vi "Write ID.vi"(8 "error in (no error)":errorcluster, 10 "ID":u8, 11 "Channel in":refnum<class "Channel.lvclass">) -> (0 "error out":errorcluster, 3 "Channel out":refnum<class "Channel.lvclass">)   [LabVIEW 2018, in "Channel.lvclass"]
uses:
  Channel.lvclass
  Channel.lvclass/Channel.ctl
  Save Image/Save Image.lvclass/Save Image.ctl
  Save Image/Save Image.lvclass
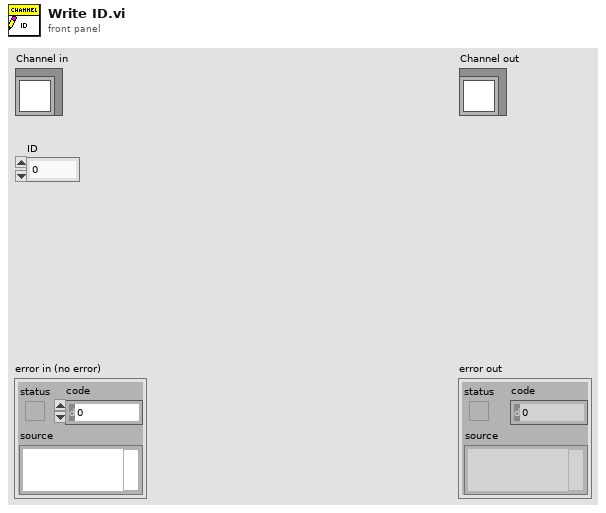
[diagram p1: front panel]
types:
  T1 = cluster{"COMNENT":string, "OBSTYPE":string, "ACSVRSN":string, "CHANNEL":u16, "LAST_IMG_NAME":string, "NIGHTDIR":string}
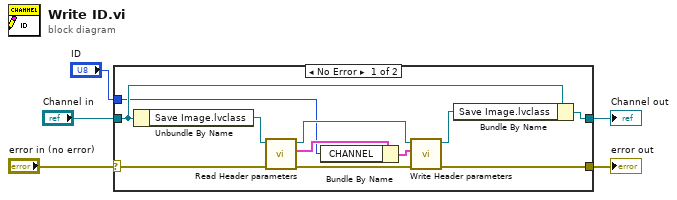
[diagram p0: block diagram]
diagram:
  n1 = case shown="No Error" "error in (no error)" {
    selector: "error in (no error)" -> [w13 w17]
    tunnel: [w11 w17] -> w4
    tunnel: [w15 w18] -> w2
    tunnel: "Channel in" -> [w16 w18]
    tunnel: "ID" -> [w6 _]
    frame No Error {
      n2 = Unbundle By Name(w16) -> ("Save Image.lvclass"=w14:refnum<class "Save Image.lvclass">)
      n3 = call "Read Header parameters.vi"("error in (no error)"=w13, "Save Image in"=w14) -> ("error out"=w12:errorcluster, "Header parameters"=w8:T1, "Save Image out"=w9:refnum<class "Save Image.lvclass">)  [unwired: 7 in]
      n4 = Bundle By Name(cluster=w8, "CHANNEL"=w6) -> (w7:T1)
      n5 = call "Write Header parameters.vi"("error in (no error)"=w12, "Header parameters"=w7, "Save Image in"=w9) -> ("error out"=w11:errorcluster, "Save Image out"=w10:refnum<class "Save Image.lvclass">)  [unwired: 7 in]
      n6 = Bundle By Name(cluster=w16, "Save Image.lvclass"=w10) -> (w15:refnum<class "Channel.lvclass">)
    }
    frame Error {
    }
  }
  "error out" <- w4
  "Channel out" <- w2
